vi "To Binary.vi"(6 "byte order":T1(ring), 8 "error in (no error)":errorcluster, 11 "Type in":refnum<class "Abs_Waveform.lvclass">) -> (0 "error out":errorcluster, 2 "Binary":string, 3 "Type out":refnum<class "Abs_Waveform.lvclass">)   [LabVIEW 2021, in "Abs_Waveform.lvclass"]
uses:
  Abs_Waveform.lvclass
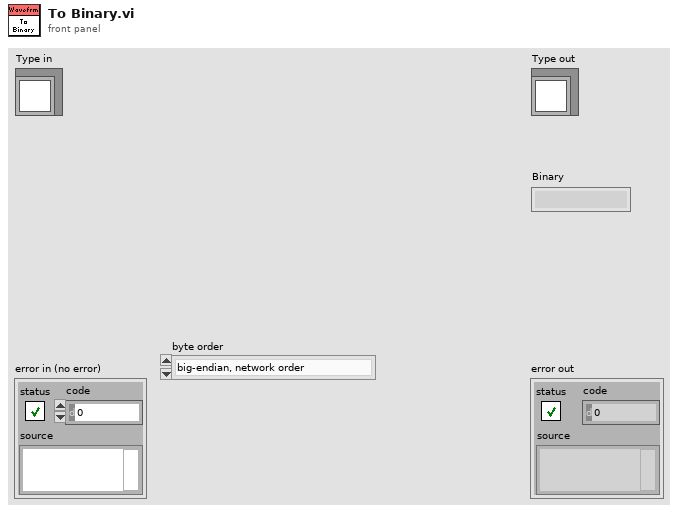
[diagram p1: front panel]
types:
  T1 = enum16{"big-endian, network order", "native, host order", "little-endian"}
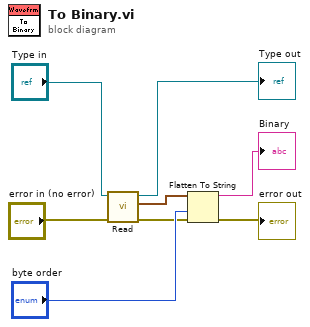
[diagram p0: block diagram]
diagram:
  n1 = call-dynamic "Read.vi"("error in (no error)"="error in (no error)", "Abs_Waveform in"="Type in") -> ("error out"=w4:errorcluster, "Waveform"=w6:waveform(dbl), "Abs_Waveform out"=→"Type out":refnum<class "Abs_Waveform.lvclass">)  [unwired: 7 in]
  n2 = Flatten To String(anything=w6, byte order (0:big-endian, network order)="byte order", error in (no error)=w4) -> (data string=→"Binary":string, error out=→"error out":errorcluster)  [unwired: 1 in, 1 out]
